vi "DAQ_Digital Pulse Gen Configure and Generate.vi"(0 "DAQmx Task In":refnum<k21>, 5 "Digital Pulse Settings":T2={"High Time (s)"=0.001, "Low Time (s)"=2e-06, "Number of Pulses"=1} {"Low Time (s)" format="%.2p"; "High Time (s)" format="%.2p"}, 11 "error in":errorcluster) -> (4 "DAQmx Task Out":refnum<k21>, 6 "Actual Pulse Settings":T1 {"Low Time (s)" format="%.2p"; "High Time (s)" format="%.2p"; "Generation Time (s)" format="%.2p"}, 15 "error out":errorcluster)   [LabVIEW 2021, in "DAQ_Digital Pulse Generation.lvlib"]
doc: "Configure and Generate Digital pulses in the configured terminal using Counters"
uses:
  DAQ_Digital Pulse Generation.lvlib
  Typedefs/Digital Pulse Settings.ctl
  Typedefs/Actual Pulse Settings.ctl
  <vilib>/DAQmx/configure/timing.llb/DAQmx Timing (Implicit).vi
  <resource>/objmgr/daqmx.rc
panel:
  out "Timebase Frequency (Hz)":dbl format="%.2p"
  # "Outputs"
  # "Inputs"
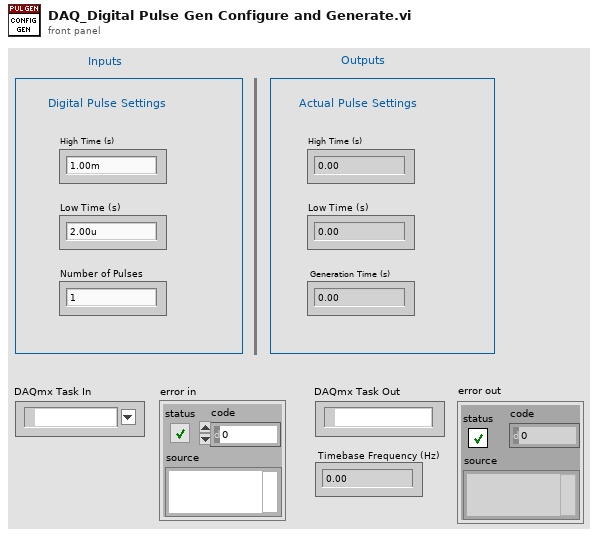
[diagram p1: front panel]
types:
  T1 = typedef "DAQ_Digital Pulse Generation.lvlib/Actual Pulse Settings.ctl" = cluster{"High Time (s)":dbl, "Low Time (s)":dbl, "Generation Time (s)":dbl}
  T2 = typedef "DAQ_Digital Pulse Generation.lvlib/Digital Pulse Settings.ctl" = cluster{"High Time (s)":dbl, "Low Time (s)":dbl, "Number of Pulses":i32}
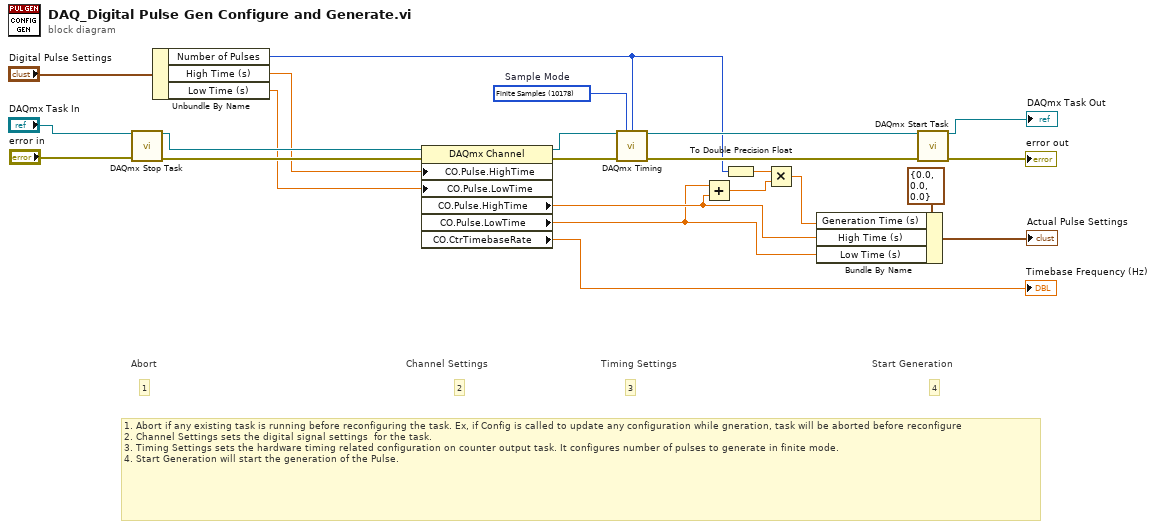
[diagram p0: block diagram]
diagram:
  w19 = 10178 items=["Finite Samples"=10178, "Continuous Samples"=10123, "Hardware Timed Single Point"=12522]  # Sample Mode
  # "1"
  # "4"
  # "3"
  # "2"
  # "Abort"
  # "1. Abort if any existing task is running before reconfiguring the task. Ex, if Config is called to update any configuration while gneration, task will be aborted before reconfigure\n2. Channel Settings sets the digital signal settings  for the task.\n3. Timing Settings sets the hardware timing related configuration on counter output task. It configures number of pulses to generate in finite mode.\n4. Start Generation will start the generation of the Pulse."
  # "Start Generation"
  # "Timing Settings"
  # "Channel Settings"
  n1 = call <vilib>:"DAQmx Stop Task.vi"("task/channels in"="DAQmx Task In", "error in"="error in") -> ("task out"=w14:refnum<k21>, "error out"=w13:errorcluster)  [unwired: 12 in]
  n2 = Unbundle By Name("Digital Pulse Settings") -> ("Number of Pulses"=w2:i32, "High Time (s)"=w7:dbl, "Low Time (s)"=w6:dbl)
  n3 = property class="DAQmx Channel"(reference=w14, error in=w13, "CO.Pulse.HighTime"=w7, "CO.Pulse.LowTime"=w6) -> (reference out=w22:refnum<k21>, error out=w23:errorcluster, "CO.Pulse.HighTime"=w5:dbl, "CO.Pulse.LowTime"=w4:dbl, "CO.CtrTimebaseRate"=→"Timebase Frequency (Hz)":dbl)
  n4 = call-poly <vilib>:"DAQmx Timing.vi"("task/channels in"=w22, "sample mode"=w19, "samples per channel"=w2, "error in"=w23) -> ("task out"=w12:refnum<k21>, "error out"=w21:errorcluster)  [unwired: 10 in]
  n5 = Add(x=w4, y=w5) -> (x+y=w3:dbl)
  n6 = To Double Precision Float(number=w2) -> (double precision float=w8:dbl)
  n7 = Multiply(x=w8, y=w3) -> (x*y=w9:dbl)
  n8 = Bundle By Name(cluster=T1 {"High Time (s)"=0.0, "Low Time (s)"=0.0, "Generation Time (s)"=0.0} ("Actual Pulse Settings"), "Generation Time (s)"=w9, "High Time (s)"=w5, "Low Time (s)"=w4) -> (→"Actual Pulse Settings":T1)
  n9 = call <vilib>:"DAQmx Start Task.vi"("task/channels in"=w12, "error in"=w21) -> ("task out"=→"DAQmx Task Out":refnum<k21>, "error out"=→"error out":errorcluster)  [unwired: 12 in]
